vi "Const frame w keyword.vi"() -> (3 "Const frame w keyword":string[](array[string]))   [LabVIEW 2018, in "Frame Analizer.lvclass"]
uses:
  Frame Analizer.lvclass
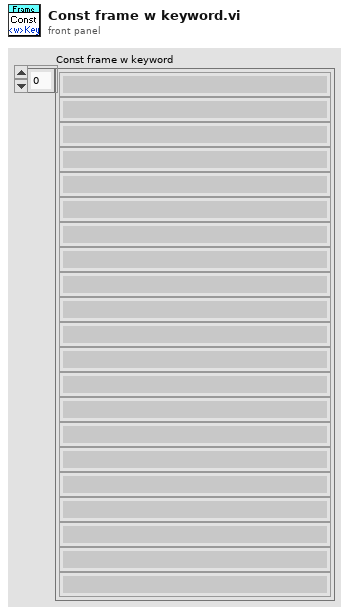
[diagram p1: front panel]
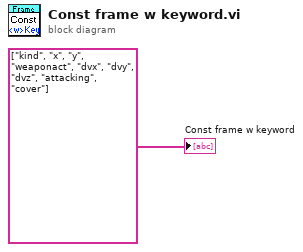
[diagram p0: block diagram]
diagram:
  "Const frame w keyword" <- string[] ["kind", "x", "y", "weaponact", "dvx", "dvy", "dvz", "attacking", "cover"]
